vi "FM Demodulation LabVIEW 2015 - NI Verified.vi"() -> ()   [LabVIEW 2015]
uses:
  <instrlib>/niUSRP/niUSRP Fetch Rx Data (CDB Cluster).vi
  <vilib>/addons/Modulation/niAMT.lvlib
panel:
  in  "Device Names":refnum<k15>
  out "FM demodulated waveform":waveform(dbl)(graph)={"t0"=timestamp(1439.77066785 s since 1904-01-01), "dt"=5e-06, "Y"=[]}
  in  "Carrier Frequency":dbl=434000000.0 format="%#_6p"
  in  "Rx IQ Rate":dbl=200000.0
  out "IQ Graph":cluster{dbl[], dbl[]}(graph)
  in  "Number of Samples":i64=20480
  in  "Stop":bool
  out "Waveform Graph":dbl[][](graph)
  out "Coerced Gain":dbl=30.0 format="%#_6f"
  out "Coerced Carrier Frequency":dbl=434000000.0092859 format="%#_6p"
  out "Coerced IQ Rate":dbl=200000.0 format="%.6p"
  in  "Active Antenna":string="RX2"
  in  "RX Gain":dbl=30.0 format="%#_6f"
  # "Overview:  FM Signal acquisition and demodulation.\nRequirements: \n1. LabVIEW 2015 or compatible\n2. NI USRP 15.0\n3. Any compatible USRP device.\nInstructions:\n1. Select the proper IP Address for your USRP. \n2. Select which Rx input has the antenna.\n3. Select the desired IQ rate, Carrier Frequency, and Rx gain. These parameters will configure the receive signal.\n4. Choose the amount of desired samples\n5. Run the VI."
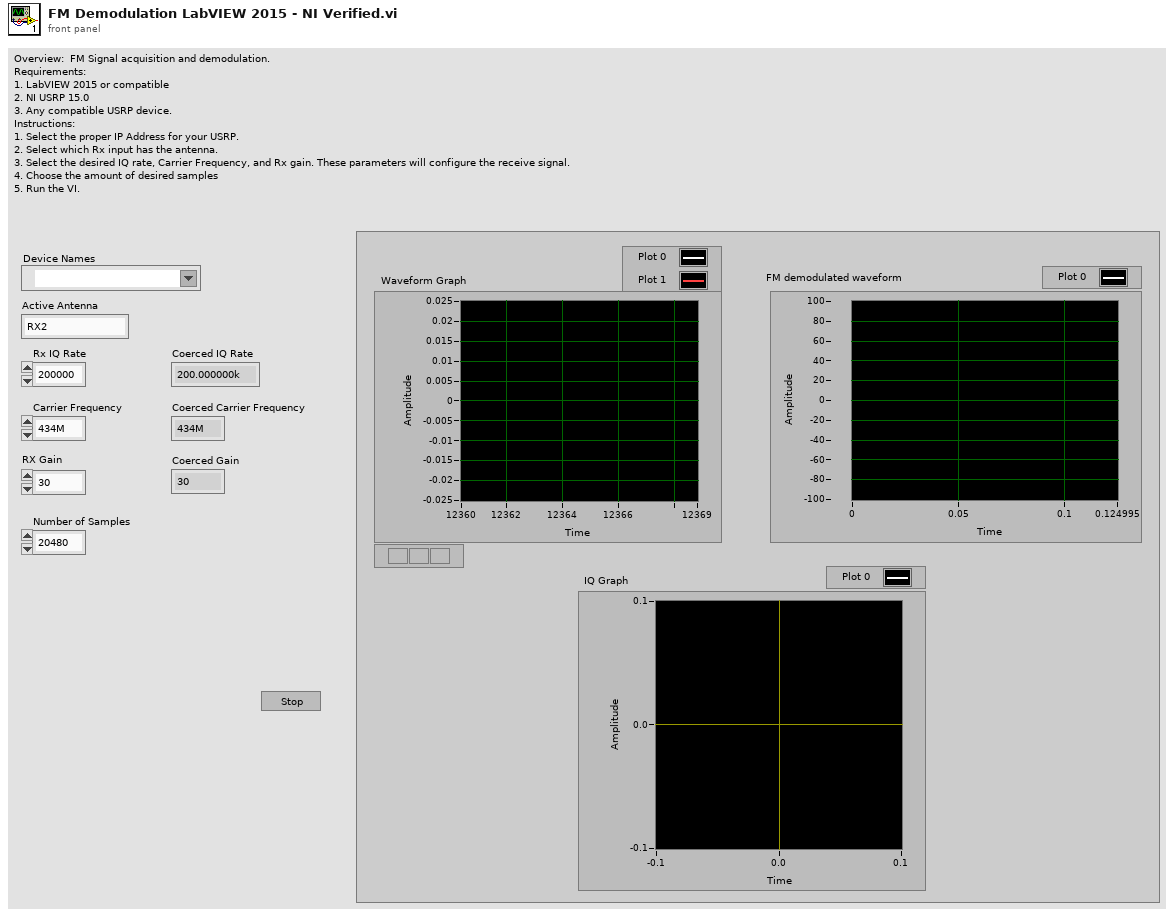
[diagram p1: front panel]
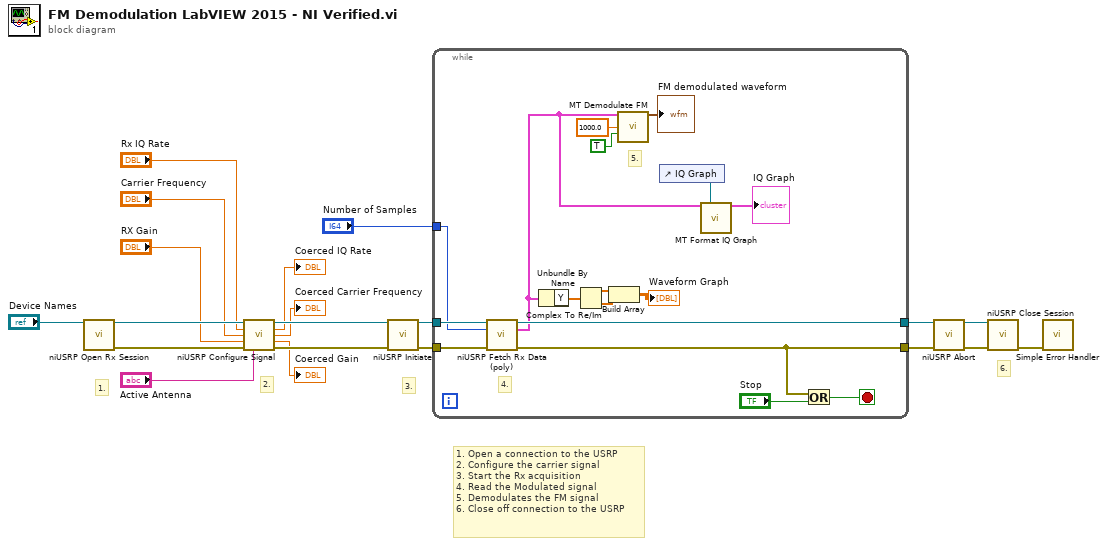
[diagram p0: block diagram]
diagram:
  # "1. Open a connection to the USRP\n2. Configure the carrier signal\n3. Start the Rx acquisition\n4. Read the Modulated signal\n5. Demodulates the FM signal\n6. Close off connection to the USRP"
  # "6."
  # "3."
  # "2."
  # "1."
  n1 = call <instrlib>:"niUSRP Open Rx Session.vi"("device names"="Device Names") -> ("session handle out"=w20:refnum<k15>, "error out"=w19:errorcluster)  [unwired: 13 in]
  n2 = call <instrlib>:"niUSRP Configure Signal.vi"("session handle"=w20, "IQ rate"="Rx IQ Rate", "carrier frequency"="Carrier Frequency", "gain"="RX Gain", "error in (no error)"=w19, "active antenna"="Active Antenna") -> ("session handle out"=w15:refnum<k15>, "coerced IQ rate"=→"Coerced IQ Rate":dbl, "coerced carrier frequency"=→"Coerced Carrier Frequency":dbl, "coerced gain"=→"Coerced Gain":dbl, "error out"=w16:errorcluster)  [unwired: 5 in]
  n3 = call <instrlib>:"niUSRP Initiate.vi"("session handle"=w15, "error in (no error)"=w16) -> ("session handle out"=w9:refnum<k15>, "error out"=w8:errorcluster)  [unwired: 12 in]
  n4 = while {
    tunnel: w9 -> [w37]
    tunnel: w8 -> [w36]
    tunnel: [w35] -> w3
    tunnel: [w27] -> w2
    tunnel: "Number of Samples" -> [w21]
    stop <- w31 stop-if-true
    # "5."
    # "4."
    n5 = call-poly <instrlib>:"niUSRP Fetch Rx Data (poly).vi"("session handle"=w37, "number of samples"=w21, "error in (no error)"=w36) -> ("session handle out"=w35:refnum<k15>, "data"=w28:cluster{"t0":dbl, "dt":dbl, "Y":cdb[]}, "error out"=w27:errorcluster)  [unwired: 9 in, 1 out]
    n6 = Unbundle By Name(w28) -> ("Y"=w29:cdb[])
    n7 = Complex To Re/Im(x + iy=w29) -> (x=w32:dbl[], y=w34:dbl[])
    n8 = Build Array(w32, w34) -> (→"Waveform Graph":dbl[][])
    n9 = call <vilib>:"MT Demodulate FM.vi"("FM modulated waveform"=w28, "FM deviation (Hz)"=1000.0, "carrier correction? (F)"=TRUE) -> ("FM demodulated waveform"=→"FM demodulated waveform":waveform(dbl))  [unwired: 10 in, 2 out]
    n10 = control-ref of="IQ Graph"() -> (w22:refnum<vi>)
    n11 = call <vilib>:"MT Format IQ Graph.vi"("IQ data (complex) in"=w28, "IQ graph reference"=w22) -> ("IQ Graph"=→"IQ Graph":cluster{dbl[], dbl[]})  [unwired: 2 in, 11 out]
    n12 = Or(x=w27, y="Stop") -> (x .or. y?=w31:bool)
  }
  n13 = call <instrlib>:"niUSRP Abort.vi"("session handle"=w3, "error in (no error)"=w2) -> ("session handle out"=w5:refnum<k15>, "error out"=w4:errorcluster)  [unwired: 12 in]
  n14 = call <instrlib>:"niUSRP Close Session.vi"("session handle"=w5, "error in (no error)"=w4) -> ("error out"=w1:errorcluster)  [unwired: 13 in]
  n15 = call <vilib>:"Simple Error Handler.vi"("error in (no error)"=w1) -> ()  [unwired: 4 in, 5 out]
